vi "createNewObject_byObject.vi"(4 "bounds":T1, 6 "location":T2, 8 "error in (no error)":errorcluster, 10 "typeToCreate":refnum<class "ICreatable.lvclass">, 11 "ownerIn":refnum<class "Generic.lvclass">) -> (0 "error out":errorcluster, 2 "created":refnum<class "ICreatable.lvclass">, 3 "ownerOut":refnum<class "Generic.lvclass">)   [LabVIEW 2023, in "TLC_Scripto.lvlib"]
uses:
  TLC_Scripto.lvlib
  Generic/Generic.lvclass
  <vilib>/Utility/miscctls.llb/LVPointTypeDef.ctl
  <vilib>/Utility/miscctls.llb/LVBoundsTypeDef.ctl
  ICreatable/ICreatable.lvclass
  Generic/Read ref.vi
  <userlib>/_OpenG.lib/error/error.llb/openg_error.lvlib
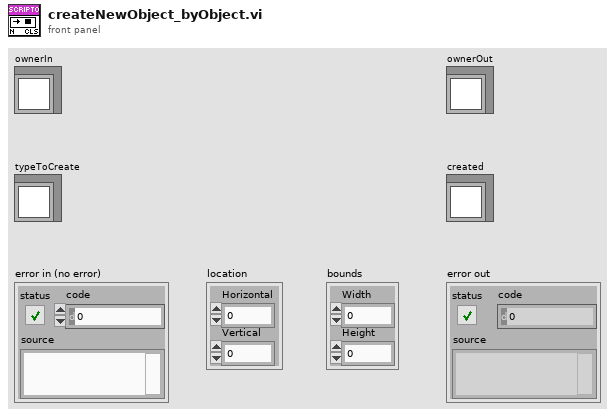
[diagram p1: front panel]
types:
  T1 = typedef "LVBoundsTypeDef.ctl" = cluster{"Width":u32, "Height":u32}
  T2 = typedef "LVPointTypeDef.ctl" = cluster{"Horizontal":i16, "Vertical":i16}
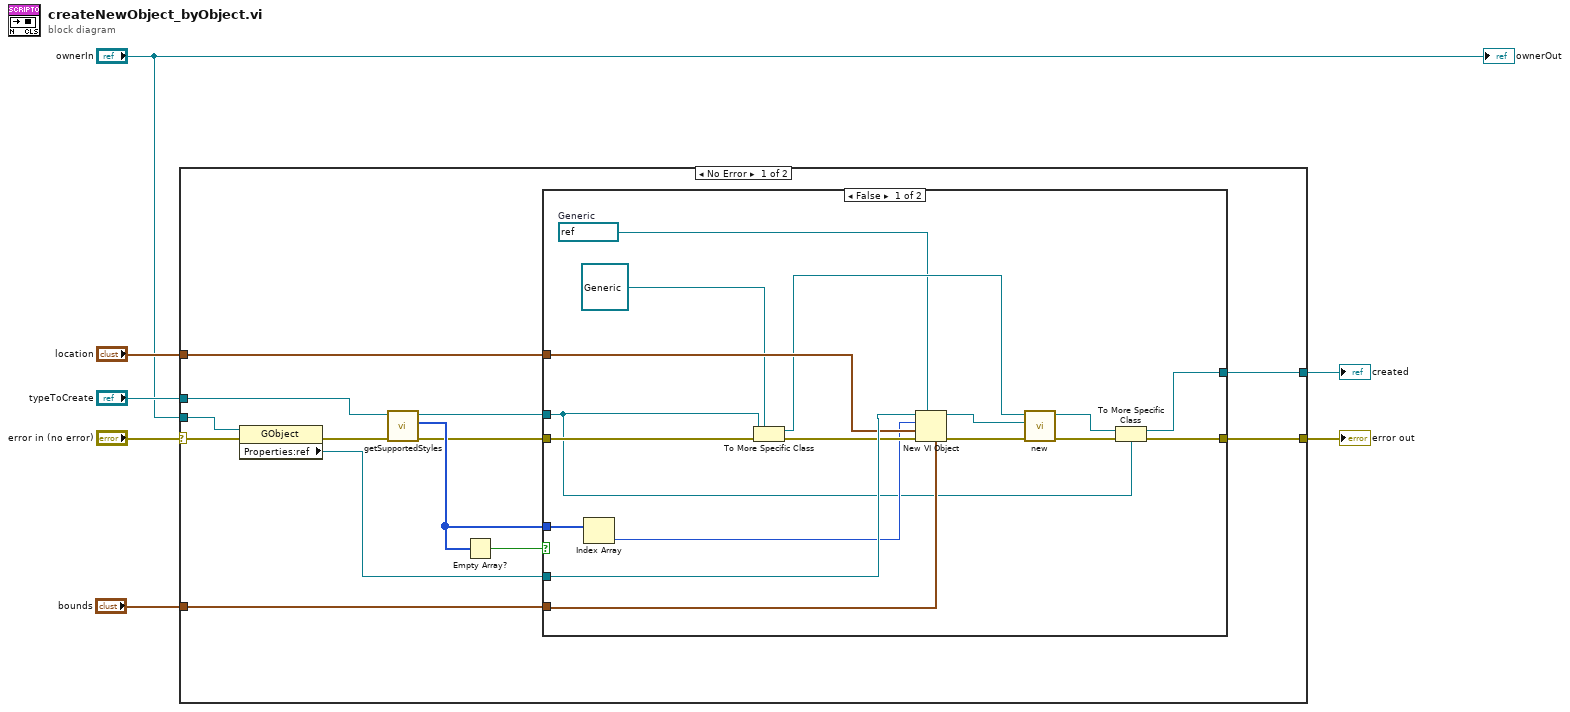
[diagram p0: block diagram]
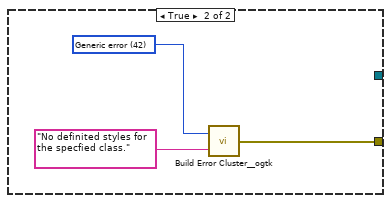
[diagram p2: hidden frame]
diagram:
  n1 = case shown="No Error" "error in (no error)" {
    selector: "error in (no error)" -> [w14 w41]
    tunnel: "ownerIn" -> [w20 _]
    tunnel: "location" -> [w18 _]
    tunnel: "bounds" -> [w17 _]
    tunnel: "typeToCreate" -> [w12 _]
    tunnel: [w16 w41] -> w4
    tunnel: [w15 _] -> w1
    frame No Error {
      n2 = property class="GObject"(reference=w20, error in=w14) -> (error out=w13:errorcluster, "Properties:ref"=w19:refnum<vi>)  [unwired: 1 out]
      n3 = call-dynamic "getSupportedStyles.vi"("error in (no error)"=w13, "ICreatable in"=w12) -> ("error out"=w8:errorcluster, "styles"=w10:i32[], "ICreatable out"=w9:refnum<class "ICreatable.lvclass">)  [unwired: 7 in]
      n4 = Empty Array?(array=w10) -> (empty?=w11:bool)
      n5 = case shown="False" w11 {
        tunnel: w19 -> [w37 _]
        tunnel: w18 -> [w36 _]
        tunnel: w17 -> [w35 _]
        tunnel: [w24 w39] -> w16
        tunnel: [w22 _] -> w15
        tunnel: w10 -> [w32 _]
        tunnel: w9 -> [w21 _]
        tunnel: w8 -> [w30 _]
        frame False {
          w26 = refnum<vi> refnum  # Generic
          n6 = Index Array(array=w32) -> (element=w27:i32)  [unwired: 1 in]
          n7 = To More Specific Class(target class=refnum<class "Generic.lvclass"> refnum ("TLC_Scripto.lvlib:GObject"), reference=w21, error in=w30) -> (specific class reference=w31:refnum<class "Generic.lvclass">, error out=w28:errorcluster)
          n8 = New VI Object(vi object class=w26, owner refnum=w37, style=w27, position/next to=w36, 4:w35, 8:w28) -> (object refnum=w33:refnum<vi>, 0:w34:errorcluster)  [unwired: 2 in]
          n9 = call-dynamic "new.vi"("Error In"=w34, "ref"=w33, "Generic In"=w31) -> ("Error Out"=w25:errorcluster, "Generic Out"=w23:refnum<class "Generic.lvclass">)  [unwired: 7 in]
          n10 = To More Specific Class(target class=w21, reference=w23, error in=w25) -> (specific class reference=w22:refnum<class "ICreatable.lvclass">, error out=w24:errorcluster)
        }
        frame True {
          w40 = 42 items=["No error", "Argument error", "Memory is full", "Out of zone", "End of file", "File already open", "Generic file I/O error", "File not found", "File permission error", "Disk is full", "Duplicate path", "Too many files open", "System feature not enabled", "Resource file not found", "Cannot add resource", "Resource not found", "Image not found", "Image memory error", "Pen does not exist", "Config type invalid", "Config token not found", "Config parse error", "Config memory error", "Bad external code format", "Bad external code offset", "External code not present", "Null window", "Destroy window error", "Null menu", "Print aborted", "Bad print record", "Print driver error", "Windows error during printing", "Memory error during printing", "Print dialog error", "Generic print error", "Invalid device refnum", "Device not found", "Device parameter error", "Device unit error", "Cannot open device", "Device call aborted", "Generic error", "Cancelled by user", "Object ID too low", "Object ID too high", "Object not in heap", "Unknown heap", "Unknown object (invalid DefProc)", "Unknown object (DefProc not in table)", "Message out of range", "Invalid (null) method", "Unknown message", "Manager call not supported", "Bad address", "Network operation in progress", "Network operation timed out", "Connection is busy", "Network attribute not supported", "Network error", "Address in use", "System out of memory", "Connection aborted", "Connection refused", "Not connected", "Already connected", "Connection closed", "Initialization error (interapplication manager)", "Bad occurrence", "Wait on unbound occurrence handler", "Occurrence queue overflow", "Datalog type conflict", "Unused", "Unrecognized type (interapplication manager)", "Memory corrupt", "Failed to make temporary DLL", "Old CIN version", "Drag socket not found", "Failed to load drop-object", "Failed to register OLE object", "Failed to release OLE object", "Format specifier type mismatch", "Unknown format specifier", "Too few format specifiers", "Too many format specifiers", "Scan failed", "Newer CIN version", "Error converting to variant", "Runtime menu error", "Password tampered", "Variant attribute not found", "Incompatible variant data type", "Event data is not available", "Event Store is not present", "Occurrence is not found", "Event Queue is not created", "Event info is not available", "Refnum passed is NULL", "Error retrieving Class GUID", "Error retrieving CoClass GUID", "Error retrieving TypeLib GUID.", "Bad built application magic bytes.", "Specific driver is different from the specific driver associated with the Logical Name.", "There is no session opened to the class driver.", "Max Error", "MAX - Error with config objects", "MAX - Error loading configuration", "MAX - Group not supported"]
          n11 = call <userlib>:"Build Error Cluster__ogtk.vi"("String to Prepend to source (\"\")"="No definited styles for the specfied class." ("format string"), "code"=w40) -> ("error out"=w39:errorcluster)
        }
      }
    }
    frame Error {
    }
  }
  "error out" <- w4
  "created" <- w1
  "ownerOut" <- "ownerIn"
